vi "UserEnterRange.vi"(0 "Max Entry":i32) -> (2 "Begin Out":i32, 3 "End Out":i32, 4 "Canceled?":bool)   [LabVIEW 2013]
panel:
  in  "Cancel":bool
  in  "Done":bool
  in  "End":i32 min=1 max=1
  in  "Begin":i32 min=1 max=6
  # "Enter the rows to delete (inclusive):"
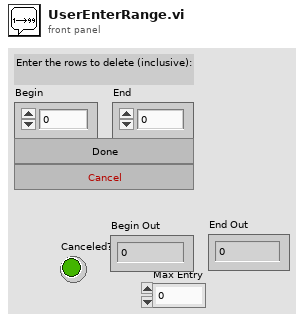
[diagram p1: front panel]
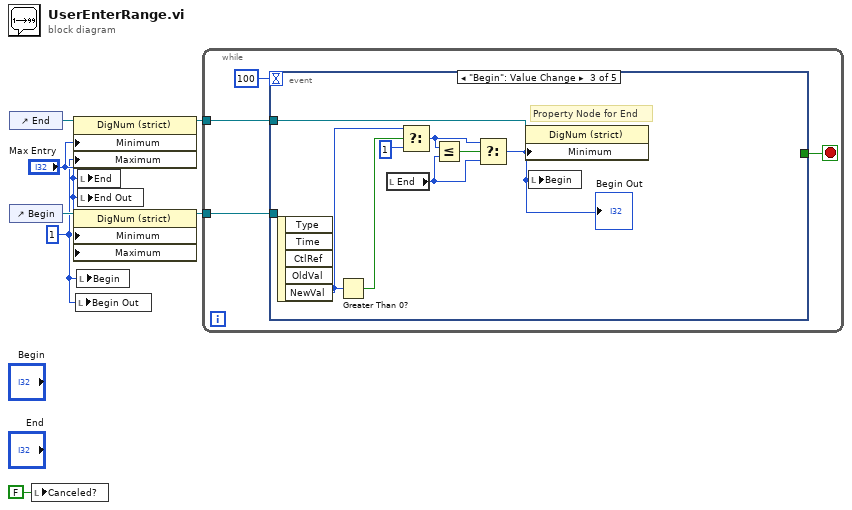
[diagram p0: block diagram]
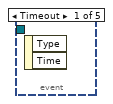
[diagram p2: hidden frame]
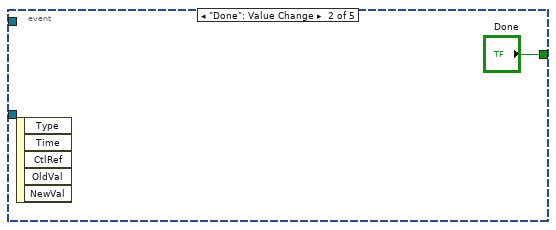
[diagram p3: hidden frame]
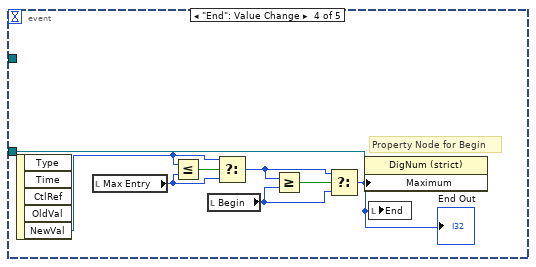
[diagram p4: hidden frame]
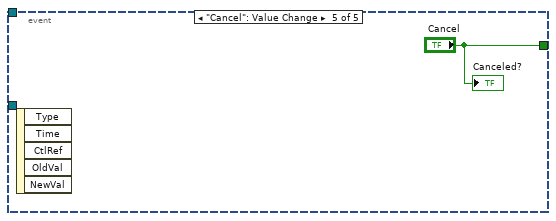
[diagram p5: hidden frame]
diagram:
  w1 = 1
  n1 = control-ref of="End"() -> (w6:refnum<vi>)
  n2 = control-ref of="Begin"() -> (w7:refnum<vi>)
  n3 = local write "Canceled?"(FALSE ("Canceled")) -> ()
  n4 = property on="Property Node" class="DigNum (strict)"(reference=w6, "Minimum"="Max Entry", "Maximum"=w1) -> (reference out=w5:refnum<vi>)  [unwired: 1 in, 1 out]
  n5 = property on="Property Node" class="DigNum (strict)"(reference=w7, "Minimum"=w1, "Maximum"="Max Entry") -> (reference out=w4:refnum<vi>)  [unwired: 1 in, 1 out]
  n6 = local write "Begin Out"(w1) -> ()
  n7 = local write "Begin"(w1) -> ()
  n8 = local write "End"("Max Entry") -> ()
  n9 = local write "End Out"("Max Entry") -> ()
  n10 = while {
    tunnel: w5 -> [w9]
    tunnel: w4 -> [w8]
    stop <- w11 stop-if-true
    n11 = event shown="[2] \"Begin\": Value Change" {
      selector: _ -> [_ _ _ _ _]
      dyn-events: _ -> [_ _ _ _ _]
      timeout: 100 -> [_ _ _ _ _]
      tunnel: [_ "Done" _ _ "Cancel"] -> w11
      tunnel: w9 -> [_ _ w20 _ _]
      tunnel: w8 -> [_ _ _ w25 _]
      event Timeout {
        n12 = event-data() -> ()  [unwired: 1 in, 2 out]
      }
      event "Done": Value Change {
        n13 = event-data() -> ()  [unwired: 1 in, 5 out]
      }
      event "Begin": Value Change {
        # "Property Node for End"
        n14 = event-data() -> ("NewVal"=w19:i32)  [unwired: 1 in, 4 out]
        n15 = Greater Than 0?(x=w19) -> (x > 0?=w18:bool)
        n16 = local read "End"() -> (w14:i32)
        n17 = Select(t=w19, s=w18, f=1) -> (s? t:f=w15:i32)
        n18 = Less Or Equal?(x=w15, y=w14) -> (x <= y?=w16:bool)
        n19 = Select(t=w15, s=w16, f=w14) -> (s? t:f=w13:i32)
        "Begin Out" <- w13
        n20 = property on="Property Node" class="DigNum (strict)"(reference=w20, "Minimum"=w13) -> ()  [unwired: 1 in, 2 out]
        n21 = local write "Begin"(w13) -> ()
      }
      event "End": Value Change {
        # "Property Node for Begin"
        n22 = event-data() -> ("NewVal"=w23:i32)  [unwired: 1 in, 4 out]
        n23 = local read "Max Entry"() -> (w22:i32)
        n24 = Less Or Equal?(x=w23, y=w22) -> (x <= y?=w28:bool)
        n25 = local read "Begin"() -> (w24:i32)
        n26 = Select(t=w23, s=w28, f=w22) -> (s? t:f=w26:i32)
        n27 = Greater Or Equal?(x=w26, y=w24) -> (x >= y?=w27:bool)
        n28 = Select(t=w26, s=w27, f=w24) -> (s? t:f=w21:i32)
        "End Out" <- w21
        n29 = property on="Property Node" class="DigNum (strict)"(reference=w25, "Maximum"=w21) -> ()  [unwired: 1 in, 2 out]
        n30 = local write "End"(w21) -> ()
      }
      event "Cancel": Value Change {
        n31 = event-data() -> ()  [unwired: 1 in, 5 out]
        "Canceled?" <- "Cancel"
      }
    }
  }
